vi "CRLF.vi"() -> (2 "CRLF":string="\r\n")   [LabVIEW 2019, in "RESP3.lvlib"]
uses:
  RESP3.lvlib
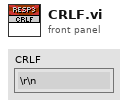
[diagram p1: front panel]
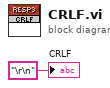
[diagram p0: block diagram]
diagram:
  "CRLF" <- "\r\n"
